vi "Update Outputs (Mark Siekmeier's conflicted copy 2013-04-30).vi"() -> ()   [LabVIEW 2012]
uses:
  <vilib>/Rock Robotics/WPI/Solenoid/WPI_SolenoidValue.ctl
  <vilib>/Rock Robotics/WPI/RobotDrive/WPI_RobotDriveGetSetRefNum.vi
  Robot Global Data.vi
  <vilib>/Rock Robotics/WPI/Solenoid/WPI_SolenoidSetEnum.vi
  <vilib>/Rock Robotics/WPI/RobotDrive/WPI_RobotDriveArcadeDrive_Standard(NoSaturation).vi
panel:
  out "Gyro Angle":dbl(knob) scale=0.0..360.0
  out "Loop Time 2":u32(graph)
  out "Right Distance (ft)":dbl
  out "Left Distance (ft)":dbl
  out "Right Rate":dbl(graph)
  out "Left Rate":dbl(graph)
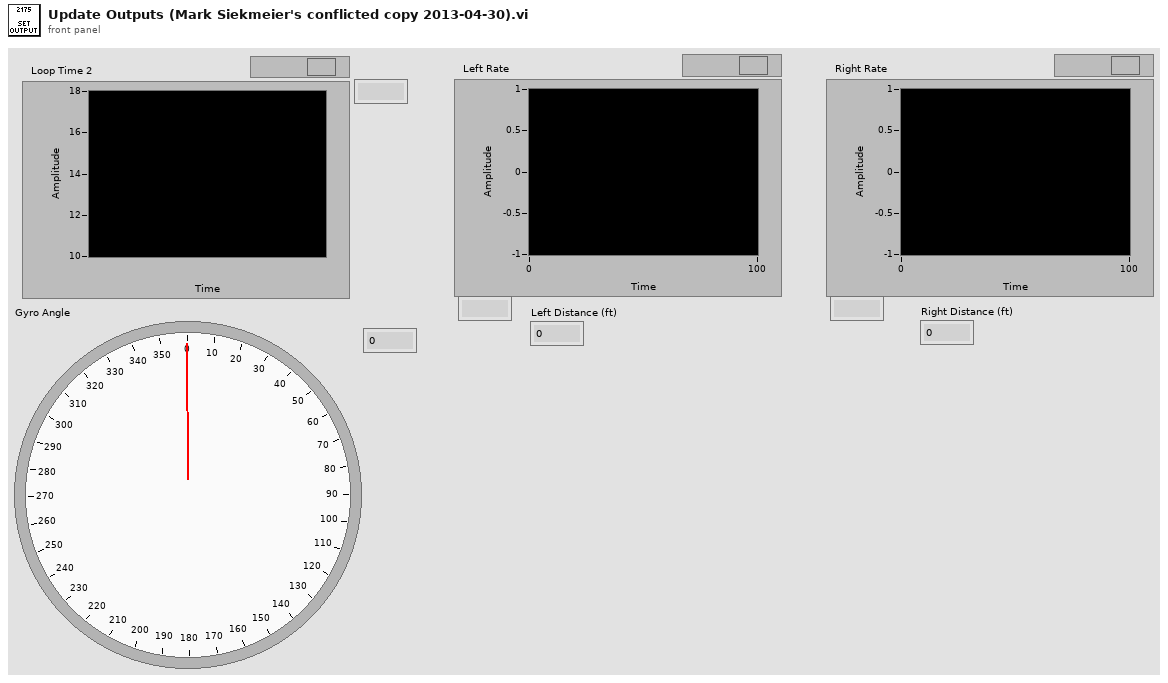
[diagram p1: front panel]
types:
  T1 = typedef "WPI_SolenoidDevRef.ctl" = cluster{"DevStatus":errorcluster, "Solenoid Module":T2, "Forward Solenoid Channel":T3, "Reverse Solenoid Channel":T3}
  T2 = typedef "FPGA_TypedefSolenoidModule.ctl" = enum16{"Solenoid Module 1", "Solenoid Module 2"}
  T3 = typedef "WPI_SolenoidChannel.ctl" = enum8{"Solenoid 1", "Solenoid 2", "Solenoid 3", "Solenoid 4", "Solenoid 5", "Solenoid 6", "Solenoid 7", "Solenoid 8", "Invalid"}
  T4 = typedef "WPI_RobotDriveDevRef.ctl" = cluster{"DevStatus":errorcluster, "Motors[]":T5[], "Square Inputs":bool, "Max Output":dbl, "Isochronous":bool}
  T5 = typedef "WPI_MotorControlDeviceRef.ctl" = cluster{"DeviceStatus":errorcluster, "Type":enum16{"PWM", "CAN"}, "PWM":cluster{"Digital Module":T6, "PWM Channel":T7, "DeadBand":T8}, "CAN":cluster{"Device Number":u8, "Control Mode":T9, "Semaphore":T10, "Max Vout":dbl}, "Invert":bool, "TransformRef":T11, "InvTransformRef":T11}
  T6 = typedef "FPGA_TypedefDigitalModule.ctl" = enum16{"Digital Module 1", "Digital Module 2"}
  T7 = typedef "FPGA_DIOPWMChannel.ctl" = enum8{"PWM 1", "PWM 2", "PWM 3", "PWM 4", "PWM 5", "PWM 6", "PWM 7", "PWM 8", "PWM 9", "PWM 10", "Invalid"}
  T8 = typedef "WPI_PWMDeadband.ctl" = cluster{"Name":string, "maxPositivePwm":i32, "minPositivePwm":i32, "centerPwm":i32, "maxNegativePwm":i32, "minNegativePwm":i32, "angularRange":u16}
  T9 = typedef "WPI_CANJaguar_ControlMode.ctl" = enum8{"Percent VBus", "Current", "Speed", "Position", "Voltage"}
  T10 = typedef "Semaphore RefNum" = refnum<k1>
  T11 = typedef "WPI_PWMTransform_ConPane.ctl" = refnum<vi>
  T12 = typedef "WPI_DigitalInputDevRef.ctl" = cluster{"DevStatus":errorcluster, "DIO Channel":T13, "Digital Module":T6}
  T13 = typedef "FPGA_DIOChannel.ctl" = enum8{"DIO 1", "DIO 2", "DIO 3", "DIO 4", "DIO 5", "DIO 6", "DIO 7", "DIO 8", "DIO 9", "DIO 10", "DIO 11", "DIO 12", "DIO 13", "DIO 14", "Invalid"}
  T14 = typedef "WPI_EncoderDevRef.ctl" = cluster{"DevStatus":errorcluster, "EncoderIndex":T15, "CounterIndex":T16, "DistancePerCount":dbl, "Decoding Type":T17}
  T15 = typedef "FPGA_EncoderIdx.ctl" = enum8{"Enc 0", "Enc 1", "Enc 2", "Enc 3", "Invalid"}
  T16 = typedef "FPGA_CounterCtrSystemIndex.ctl" = enum8{"Ctr 0", "Ctr 1", "Ctr 2", "Ctr 3", "Ctr 4", "Ctr 5", "Ctr 6", "Ctr 7", "Invalid"}
  T17 = typedef "WPI_EncoderType.ctl" = enum16{"1x", "2x", "4x"}
  T18 = typedef "WPI_SolenoidValue.ctl" = enum16{"Off", "On", "Forward", "Reverse"}
  T19 = typedef "WPI_GyroDevRef.ctl" = cluster{"DevStatus":errorcluster, "Analog Module":T20, "Analog Channel":T21, "Offset":dbl, "Gain (VoltsPerDegree/Second)":dbl}
  T20 = typedef "FPGA_TypedefAnalogModule.ctl" = enum16{"Analog Module 1", "Analog Module 2"}
  T21 = typedef "FPGA_AIChannel.ctl" = enum8{"AI 1", "AI 2", "AI 3", "AI 4", "AI 5", "AI 6", "AI 7", "AI 8", "Invalid"}
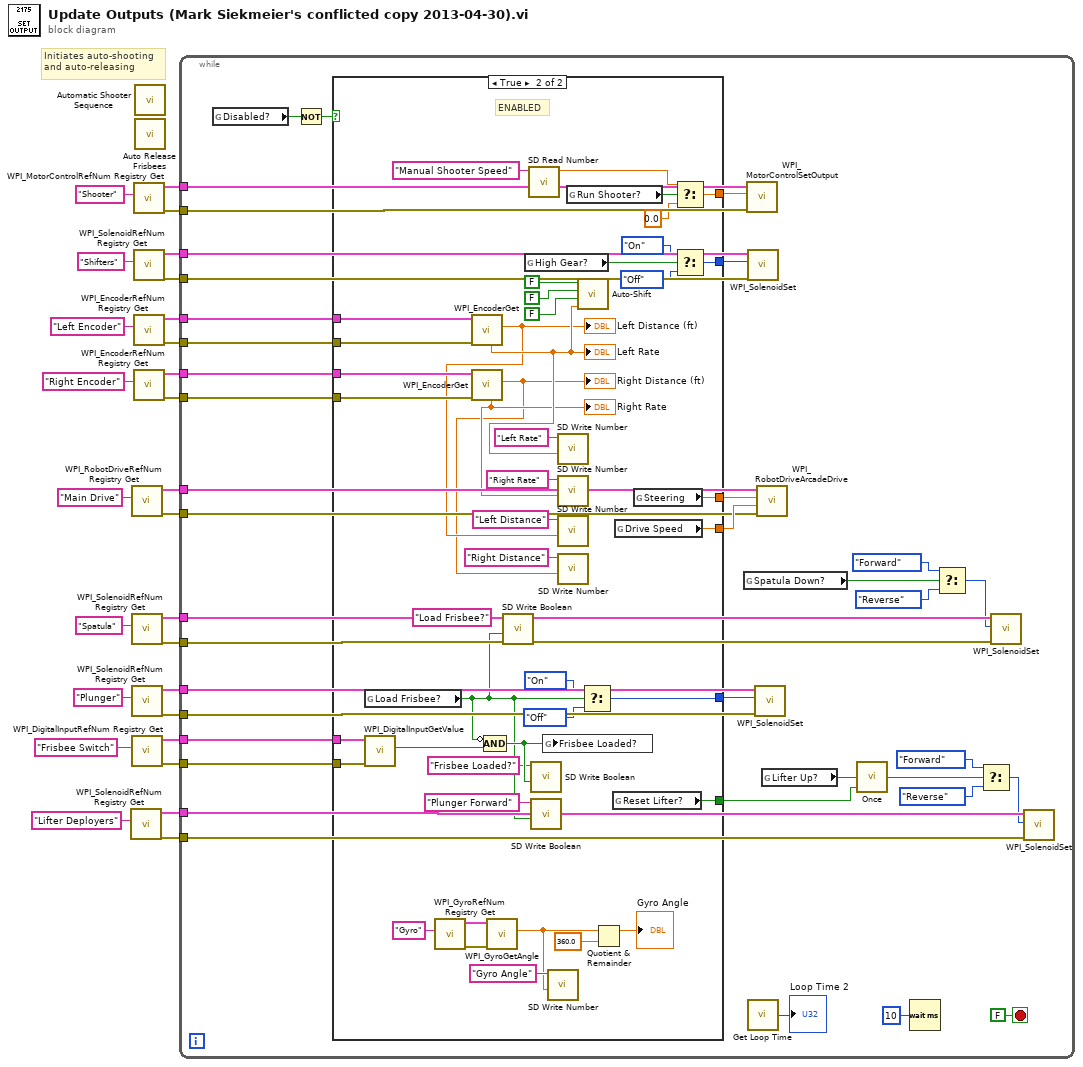
[diagram p0: block diagram]
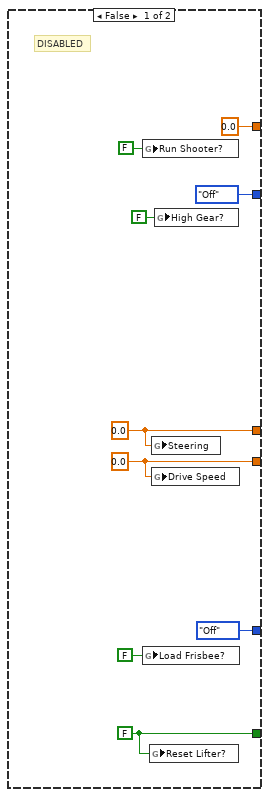
[diagram p2: hidden frame]
diagram:
  # "Initiates auto-shooting\nand auto-releasing"
  n1 = call <vilib>:"WPI_SolenoidRefNum Registry Get.vi"("refnum name"="Lifter Deployers") -> ("error out"=w1:errorcluster, "SolenoidDevRef"=w2:T1)  [unwired: 9 in]
  n2 = call <vilib>:"WPI_RobotDriveRefNum Registry Get.vi"("refnum name"="Main Drive") -> ("error out"=w22:errorcluster, "RobotDriveDevRef"=w23:T4)  [unwired: 9 in]
  n3 = call <vilib>:"WPI_SolenoidRefNum Registry Get.vi"("refnum name"="Spatula") -> ("error out"=w16:errorcluster, "SolenoidDevRef"=w17:T1)  [unwired: 9 in]
  n4 = call <vilib>:"WPI_SolenoidRefNum Registry Get.vi"("refnum name"="Plunger") -> ("error out"=w15:errorcluster, "SolenoidDevRef"=w14:T1)  [unwired: 9 in]
  n5 = call <vilib>:"WPI_DigitalInputRefNum Registry Get.vi"("refnum name"="Frisbee Switch") -> ("error out"=w4:errorcluster, "DigitalInputDevRef"=w5:T12)  [unwired: 9 in]
  n6 = call <vilib>:"WPI_MotorControlRefNum Registry Get.vi"("refnum name"="Shooter") -> ("error out"=w25:errorcluster, "MotorControlDevRef"=w26:T5)  [unwired: 9 in]
  n7 = call <vilib>:"WPI_SolenoidRefNum Registry Get.vi"("refnum name"="Shifters") -> ("error out"=w19:errorcluster, "SolenoidDevRef"=w20:T1)  [unwired: 9 in]
  n8 = call <vilib>:"WPI_EncoderRefNum Registry Get.vi"("refnum name"="Left Encoder") -> ("error out"=w10:errorcluster, "EncoderDevRef"=w11:T14)  [unwired: 9 in]
  n9 = call <vilib>:"WPI_EncoderRefNum Registry Get.vi"("refnum name"="Right Encoder") -> ("error out"=w9:errorcluster, "EncoderDevRef"=w8:T14)  [unwired: 9 in]
  n10 = call "Automatic Shooter Sequence.vi"() -> ()  [unwired: 12 in]
  n11 = call "Auto Release Frisbees.vi"() -> ()  [unwired: 12 in]
  n12 = while {
    tunnel: w26 -> [w61]
    tunnel: w25 -> [w60]
    tunnel: w23 -> [w57]
    tunnel: w22 -> [w56]
    tunnel: w20 -> [w55]
    tunnel: w19 -> [w54]
    tunnel: w17 -> [w52]
    tunnel: w16 -> [w53]
    tunnel: w14 -> [w51]
    tunnel: w15 -> [w50]
    tunnel: w11 -> [w46]
    tunnel: w10 -> [w45]
    tunnel: w8 -> [w43]
    tunnel: w9 -> [w44]
    tunnel: w5 -> [w42]
    tunnel: w4 -> [w41]
    tunnel: w2 -> [w40]
    tunnel: w1 -> [w39]
    stop <- FALSE stop-if-true
    n13 = global read "Robot Global Data.vi" "Disabled?"() -> (w63:bool)
    n14 = Not(x=w63) -> (.not. x?=w62:bool)
    n15 = case shown="True" w62 {
      tunnel: [0.0 ("Output") w103] -> w47
      tunnel: [w66 w119] -> w59
      tunnel: [w67 w111] -> w58
      tunnel: [WPI_SolenoidValue."Off" ("Value") w113] -> w49
      tunnel: [WPI_SolenoidValue."Off" ("Value") w109] -> w48
      tunnel: w46 -> [_ w107]
      tunnel: w45 -> [_ w106]
      tunnel: w43 -> [_ w100]
      tunnel: w44 -> [_ w101]
      tunnel: w42 -> [_ w99]
      tunnel: w41 -> [_ w98]
      tunnel: [w68 w94] -> w32
      frame False {
        w68 = FALSE ("High Gear?")
        w67 = 0.0 ("Drive Speed")
        w66 = 0.0 ("Steering")
        # "DISABLED"
        n16 = global write "Robot Global Data.vi" "Run Shooter?"(FALSE ("High Gear?")) -> ()
        n17 = global write "Robot Global Data.vi" "Load Frisbee?"(FALSE ("High Gear?")) -> ()
        n18 = global write "Robot Global Data.vi" "Reset Lifter?"(w68) -> ()
        n19 = global write "Robot Global Data.vi" "Steering"(w66) -> ()
        n20 = global write "Robot Global Data.vi" "Drive Speed"(w67) -> ()
        n21 = global write "Robot Global Data.vi" "High Gear?"(FALSE ("High Gear?")) -> ()
      }
      frame True {
        # "ENABLED"
        n22 = global read "Robot Global Data.vi" "Load Frisbee?"() -> (w90:bool)
        n23 = call <vilib>:"WPI_DigitalInputGetValue.vi"("error in (no error)"=w98, "DigitalInputDevRef"=w99) -> ("Value"=w97:bool)  [unwired: 7 in, 2 out]
        n24 = call <vilib>:"WPI_GyroRefNum Registry Get.vi"("refnum name"="Gyro") -> ("error out"=w80:errorcluster, "GyroDevRef"=w79:T19)  [unwired: 9 in]
        n25 = call <vilib>:"WPI_EncoderGet.vi"("error in (no error)"=w106, "EncoderDevRef"=w107) -> ("Distance"=w83:dbl, "Rate"=w85:dbl)  [unwired: 4 in, 4 out]
        "Left Rate" <- w85
        "Left Distance (ft)" <- w83
        n26 = call <vilib>:"WPI_EncoderGet.vi"("error in (no error)"=w101, "EncoderDevRef"=w100) -> ("Distance"=w82:dbl, "Rate"=w84:dbl)  [unwired: 4 in, 4 out]
        "Right Rate" <- w84
        "Right Distance (ft)" <- w82
        n27 = Compound Arithmetic op=AND(invert w90, w97) -> (w96:bool)
        n28 = call <vilib>:"WPI_GyroGetAngle.vi"("error in (no error)"=w80, "GyroDevRef"=w79) -> ("Angle"=w77:dbl)  [unwired: 6 in, 3 out]
        n29 = call <vilib>:"SD Write Boolean.vi"("Boolean"=w90, "Name"="Load Frisbee?") -> ()  [unwired: 8 in, 2 out]
        n30 = global read "Robot Global Data.vi" "High Gear?"() -> (w118:bool)
        n31 = call <vilib>:"SD Read Number.vi"("Name"="Manual Shooter Speed") -> ("Numeric"=w104:dbl)  [unwired: 8 in, 2 out]
        n32 = call <vilib>:"SD Write Boolean.vi"("Boolean"=w96, "Name"="Frisbee Loaded?") -> ()  [unwired: 8 in, 2 out]
        n33 = call <vilib>:"SD Write Boolean.vi"("Boolean"=w90, "Name"="Plunger Forward") -> ()  [unwired: 8 in, 2 out]
        n34 = global write "Robot Global Data.vi" "Frisbee Loaded?"(w96) -> ()
        n35 = call <vilib>:"SD Write Number.vi"("Numeric"=w77, "Name"="Gyro Angle") -> ()  [unwired: 8 in, 2 out]
        n36 = call <vilib>:"SD Write Number.vi"("Numeric"=w85, "Name"="Left Rate") -> ()  [unwired: 8 in, 2 out]
        n37 = call <vilib>:"SD Write Number.vi"("Numeric"=w84, "Name"="Right Rate") -> ()  [unwired: 8 in, 2 out]
        n38 = call <vilib>:"SD Write Number.vi"("Numeric"=w83, "Name"="Left Distance") -> ()  [unwired: 8 in, 2 out]
        n39 = call <vilib>:"SD Write Number.vi"("Numeric"=w82, "Name"="Right Distance") -> ()  [unwired: 8 in, 2 out]
        n40 = global read "Robot Global Data.vi" "Run Shooter?"() -> (w105:bool)
        n41 = call "Auto-Shift.vi"("Average Ft/Sec"=w85, "Coastdown Enabled?"=FALSE, "Kickdown Enabled?"=FALSE, "Upshift Enabled?"=FALSE) -> ()  [unwired: 1 in]
        n42 = Select(t=WPI_SolenoidValue."On" ("Value"), s=w90, f=WPI_SolenoidValue."Off" ("Value")) -> (s? t:f=w113:T18)
        n43 = Quotient & Remainder(x=w77, y=360.0) -> (x-y*floor(x/y)=→"Gyro Angle":dbl)  [unwired: 1 out]
        n44 = global read "Robot Global Data.vi" "Reset Lifter?"() -> (w94:bool)
        n45 = global read "Robot Global Data.vi" "Drive Speed"() -> (w111:dbl)
        n46 = global read "Robot Global Data.vi" "Steering"() -> (w119:dbl)
        n47 = Select(t=w104, s=w105, f=0.0) -> (s? t:f=w103:dbl)
        n48 = Select(t=WPI_SolenoidValue."On" ("Value"), s=w118, f=WPI_SolenoidValue."Off" ("Value")) -> (s? t:f=w109:T18)
      }
    }
    n49 = global read "Robot Global Data.vi" "Spatula Down?"() -> (w31:bool)
    n50 = call <vilib>:"WPI_MotorControlSetOutput.vi"("error in (no error)"=w60, "Output"=w47, "MotorControlDevRef"=w61) -> ()  [unwired: 6 in, 3 out]
    n51 = call-poly <vilib>:"WPI_SolenoidSet.vi"("error in (no error)"=w54, "Value"=w48, "SolenoidDevRef"=w55) -> ()  [unwired: 7 in, 2 out]
    n52 = call "Get Loop Time.vi"() -> ("Loop Time"=→"Loop Time 2":u32)  [unwired: 1 in]
    n53 = call-poly <vilib>:"WPI_SolenoidSet.vi"("error in (no error)"=w50, "Value"=w49, "SolenoidDevRef"=w51) -> ()  [unwired: 7 in, 2 out]
    n54 = call-poly <vilib>:"WPI_RobotDriveArcadeDrive.vi"("error in (no error)"=w56, "Y axis value"=w58, "X axis value"=w59, "RobotDriveDevRef"=w57) -> ()  [unwired: 5 in, 3 out]
    n55 = global read "Robot Global Data.vi" "Lifter Up?"() -> (w34:bool)
    n56 = call "Once.vi"("Reset?"=w32, "Input"=w34) -> ("Output"=w33:bool)  [unwired: 1 in]
    n57 = Wait (ms)(milliseconds to wait=u32 10) -> ()  [unwired: 1 out]
    n58 = Select(t=WPI_SolenoidValue."Forward" ("Value"), s=w31, f=WPI_SolenoidValue."Reverse" ("Value")) -> (s? t:f=w28:T18)
    n59 = Select(t=WPI_SolenoidValue."Forward" ("Value"), s=w33, f=WPI_SolenoidValue."Reverse" ("Value")) -> (s? t:f=w35:T18)
    n60 = call-poly <vilib>:"WPI_SolenoidSet.vi"("error in (no error)"=w53, "Value"=w28, "SolenoidDevRef"=w52) -> ()  [unwired: 7 in, 2 out]
    n61 = call-poly <vilib>:"WPI_SolenoidSet.vi"("error in (no error)"=w39, "Value"=w35, "SolenoidDevRef"=w40) -> ()  [unwired: 7 in, 2 out]
  }
